vi "SrvGetStatus.vi"(0 "ref in":u64, 11 "error in (no error)":errorcluster) -> (4 "ref out":u64, 6 "return type":i32, 12 "ClientsCount":i32, 13 "CpuStatus":i32(ring)=8 items=["Run"=8, "Stop"=4], 14 "ServerStatus":i32(ring)=1 items=["Stop", "Run", "Error"], 15 "error out":errorcluster)   [LabVIEW 2010, in "Snap7.lvlib"]
uses:
  Snap7.lvlib
  windows/lv_snap7.dll
panel:
  in  "var ClientsCount":i32
  in  "var CpuStatus":i32
  in  "var ServerStatus":i32
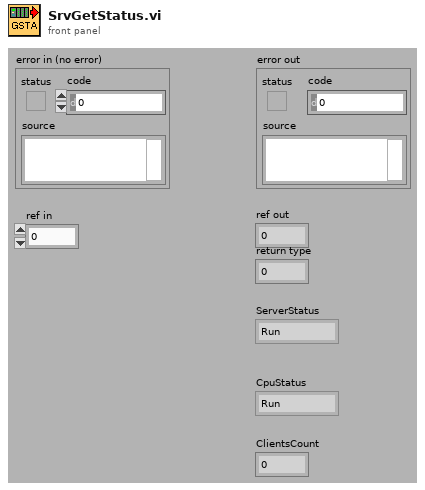
[diagram p1: front panel]
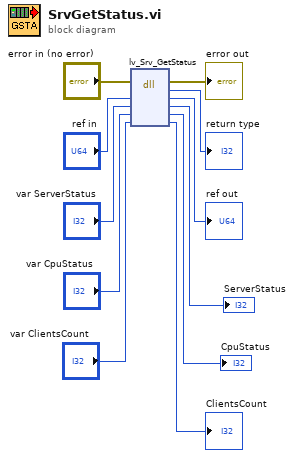
[diagram p0: block diagram]
diagram:
  n1 = dll-call lib="C:/snap7-src-1.0.0/LabVIEW/lib/windows/lv_snap7.dll" fn="lv_Srv_GetStatus"(error in="error in (no error)", "Server"="ref in", "ServerStatus"="var ServerStatus", "CpuStatus"="var CpuStatus", "ClientsCount"="var ClientsCount") -> (error out=→"error out":errorcluster, "return type"=→"return type":i32, "Server"=→"ref out":u64, "ServerStatus"=→"ServerStatus":i32, "CpuStatus"=→"CpuStatus":i32, "ClientsCount"=→"ClientsCount":i32)  [unwired: 2 in, 1 out]
